vi "Sagar C V 2X1 Multiplexer (1).vi"() -> ()   [LabVIEW 2018]
panel:
  out "Y":bool
  in  "S":bool
  in  "I0":bool
  in  "I1":bool
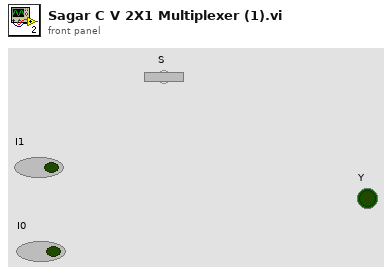
[diagram p1: front panel]
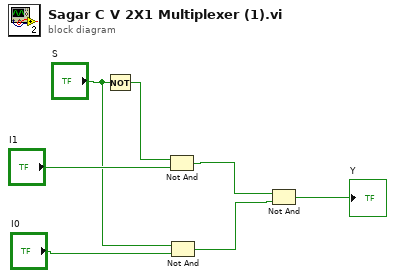
[diagram p0: block diagram]
diagram:
  n1 = Not(x="S") -> (.not. x?=w6:bool)
  n2 = Not And(1:"I1", 2:w6) -> (0:w1:bool)
  n3 = Not And(1:"I0", 2:"S") -> (0:w2:bool)
  n4 = Not And(1:w2, 2:w1) -> (0:→"Y":bool)
